vi "UI_Template_modify.vi"() -> ()   [LabVIEW 2014]
uses:
  Terminal_Global_Template_Name.vi
panel:
  in  "退出":bool
  in  "模板名称 2":string
  out "tempNo":string
  in  "修改载荷谱模板 2":string[][](table)
  in  "模板名称":string
  in  "保存修改":bool
  in  "修改载荷谱模板":string[][](table)
  # "载荷谱模板修改"
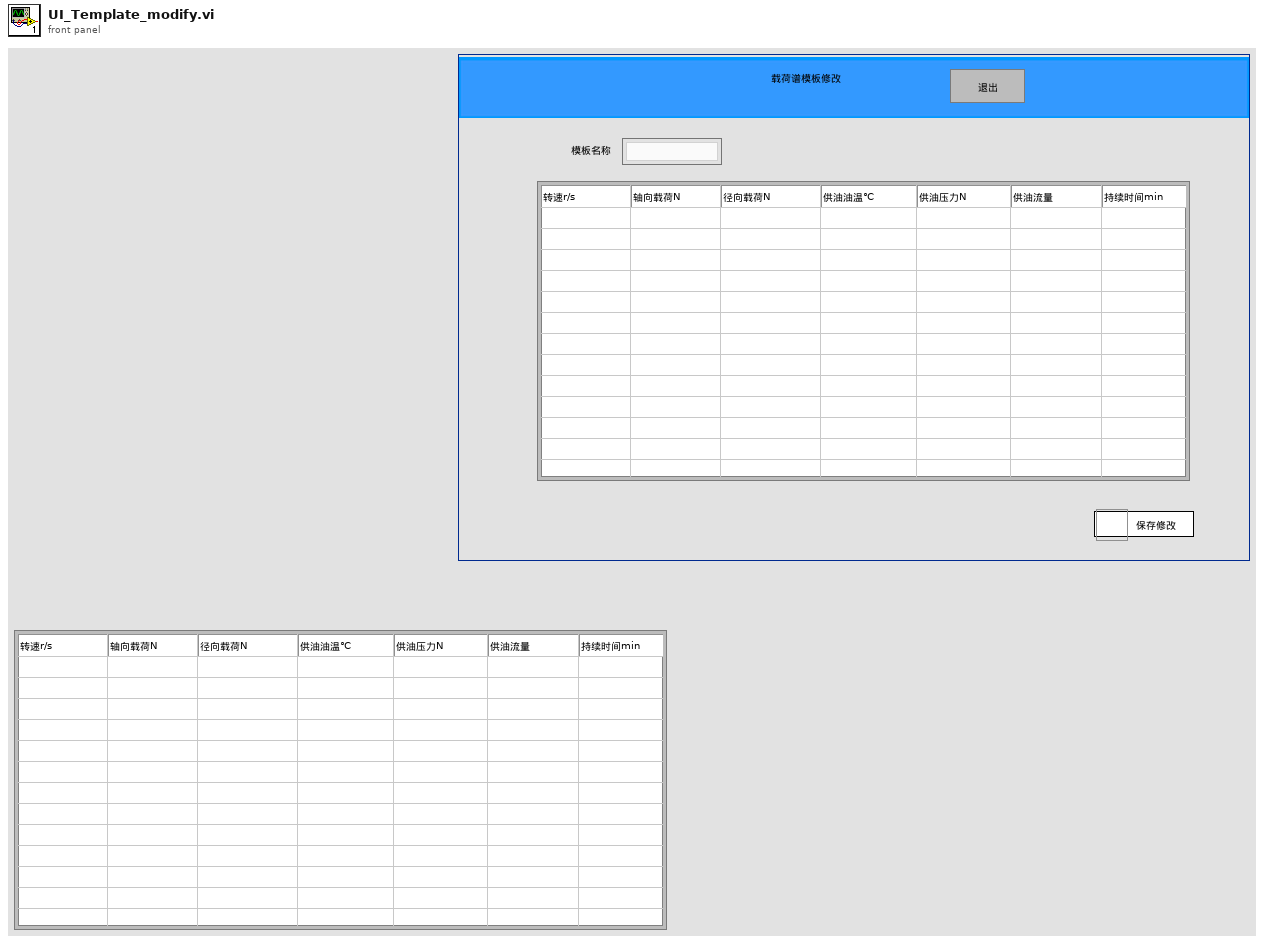
[diagram p1: front panel]
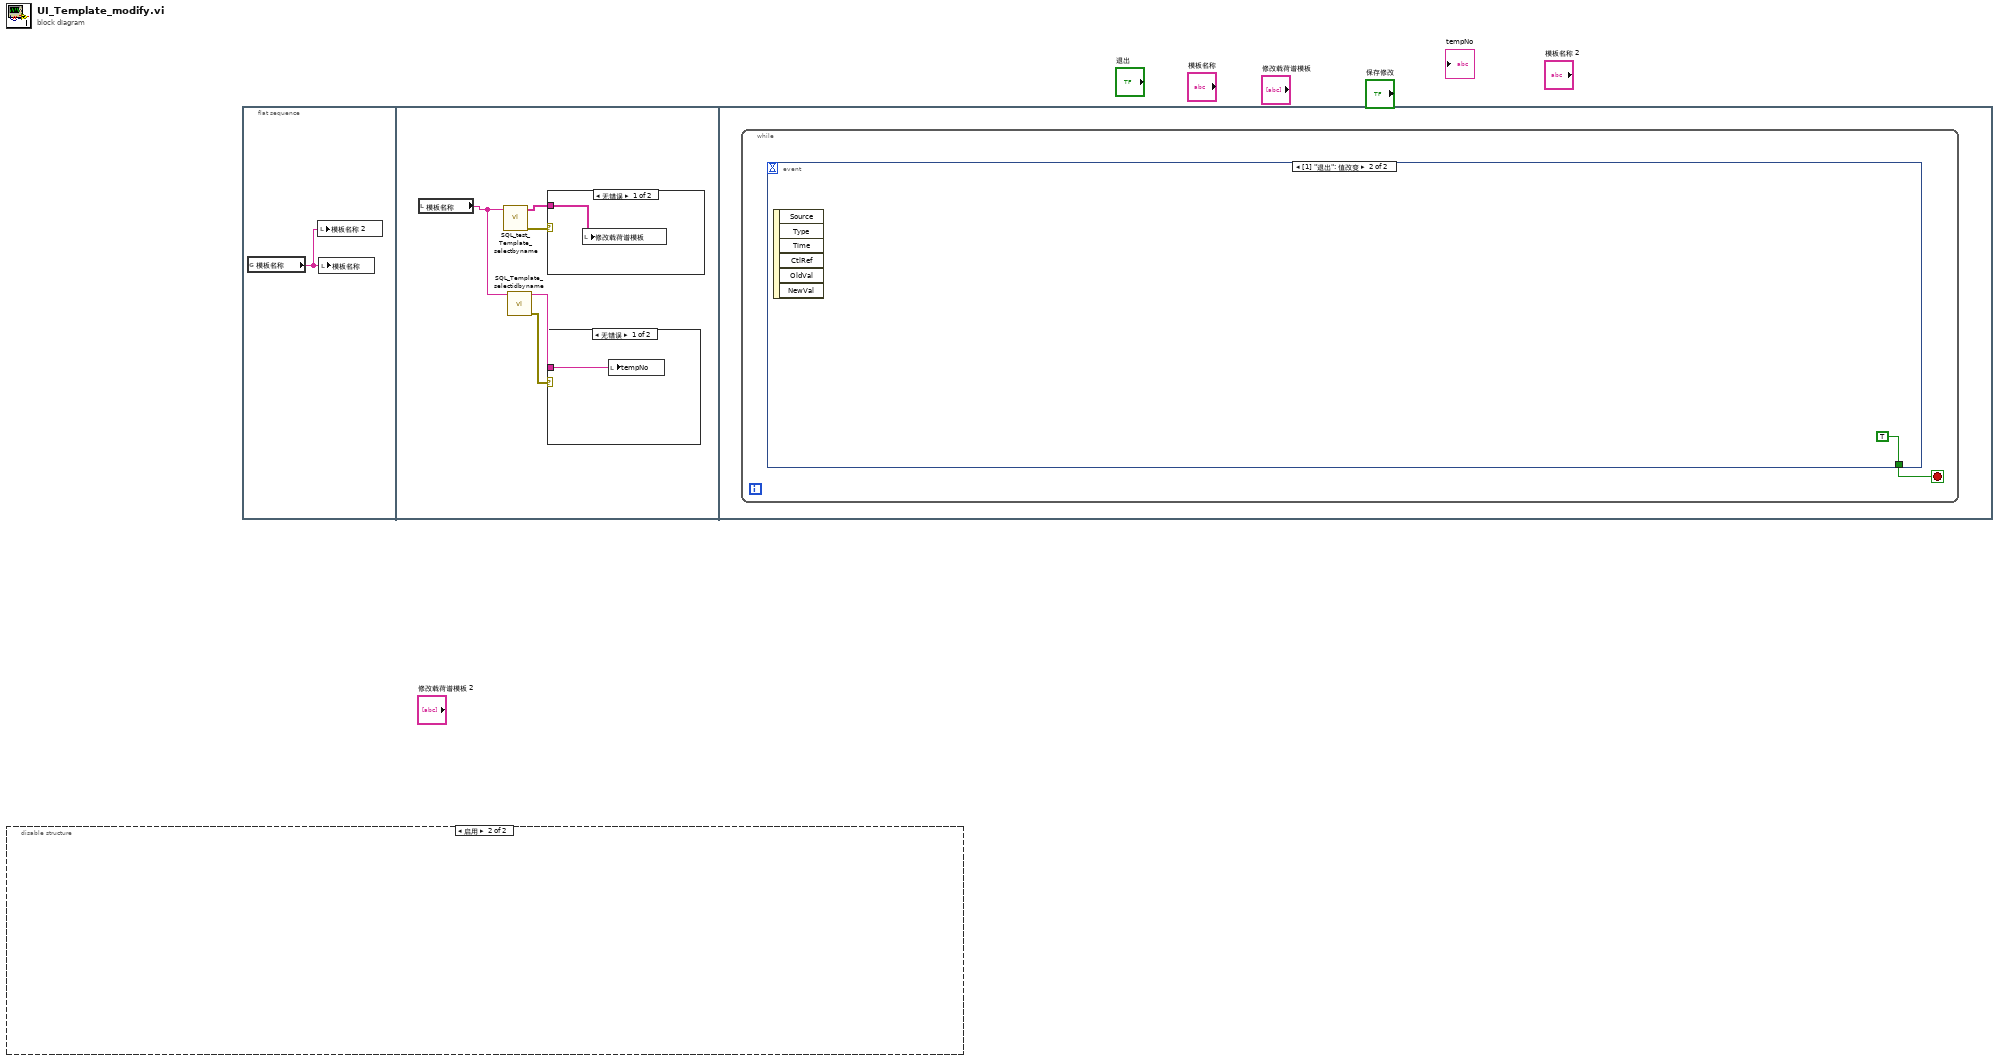
[diagram p0: block diagram]
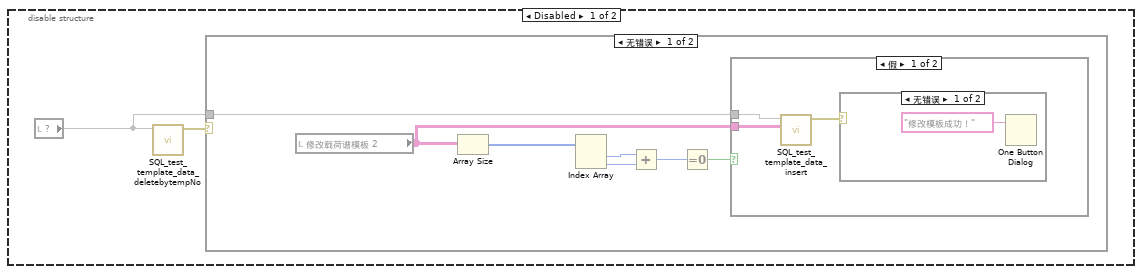
[diagram p2: hidden frame]
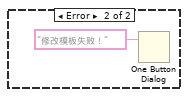
[diagram p3: hidden frame]
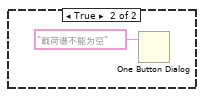
[diagram p4: hidden frame]
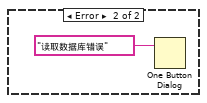
[diagram p6: hidden frame]
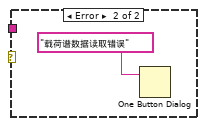
[diagram p7: hidden frame]
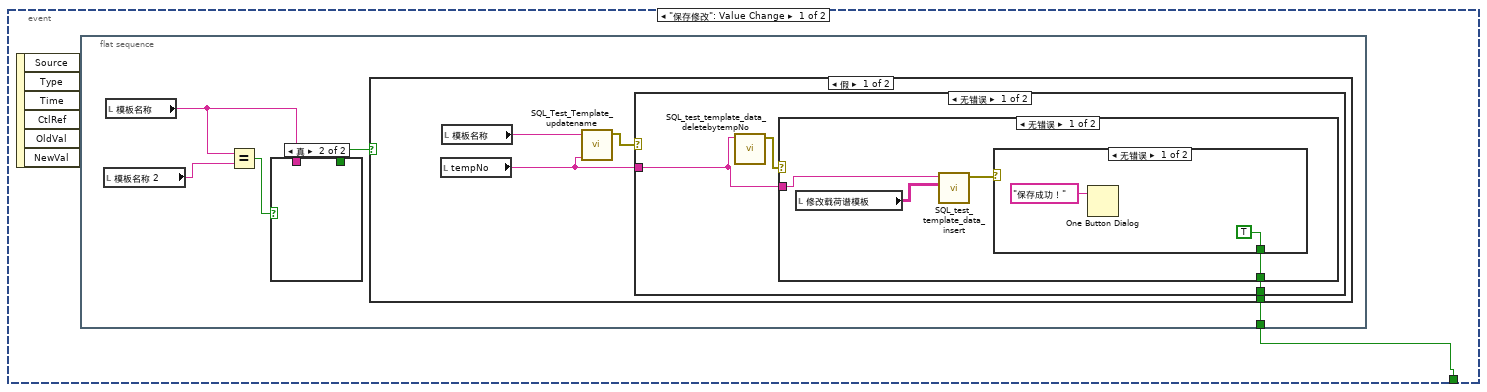
[diagram p8: hidden frame]
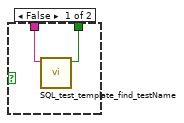
[diagram p9: hidden frame]
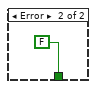
[diagram p10: hidden frame]
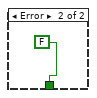
[diagram p11: hidden frame]
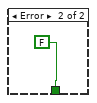
[diagram p12: hidden frame]
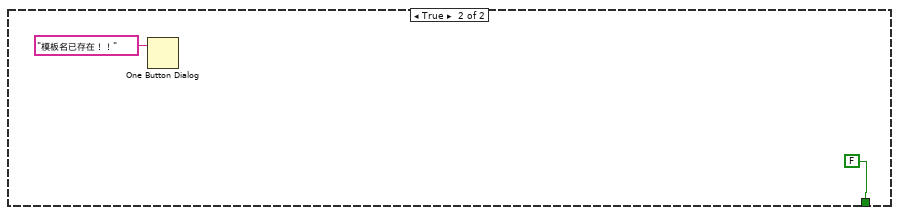
[diagram p13: hidden frame]
diagram:
  n1 = disable-structure shown="启用" {
    frame Disabled {
      n2 = local read item#-1() -> (w1)
      n3 = call "SQL_test_template_data_deletebytempNo.vi"("tempNo"=w1) -> ("error out"=w2:errorcluster)  [unwired: 10 in]
      n4 = case shown="无错误" w2 {
        tunnel: w1 -> [w3 _]
        frame No Error {
          n5 = local read "修改载荷谱模板 2"() -> (w4:string[][])
          n6 = Array Size(array=w4) -> (size(s)=w9:i32[])
          n7 = Index Array(array=w9) -> (element #1=w8:i32, element #2=w7:i32)  [unwired: 2 in]
          n8 = Add(x=w8, y=w7) -> (x+y=w6:i32)
          n9 = Equal To 0?(x=w6) -> (x = 0?=w5:bool)
          n10 = case shown="假" w5 {
            tunnel: w4 -> [w11 _]
            tunnel: w3 -> [w10 _]
            frame False {
              n11 = call "SQL_test_template_data_insert.vi"("表格控件"=w11, "tempNo"=w10) -> ("error out"=w12:errorcluster)  [unwired: 9 in]
              n12 = case shown="无错误" w12 {
                frame No Error {
                  n13 = One Button Dialog(message="修改模板成功！" ("消息")) -> ()  [unwired: 1 in, 1 out]
                }
                frame Error {
                  n14 = One Button Dialog(message="修改模板失败！" ("消息")) -> ()  [unwired: 1 in, 1 out]
                }
              }
            }
            frame True {
              n15 = One Button Dialog(message="载荷谱不能为空" ("消息")) -> ()  [unwired: 1 in, 1 out]
            }
          }
        }
        frame Error {
        }
      }
    }
    frame Enabled {
    }
  }
  n16 = flat-sequence {
    frame #0 {
      n17 = global read "Terminal_Global_Template_Name.vi" "模板名称"() -> (w16:string)
      n18 = local write "模板名称 2"(w16) -> ()
      n19 = local write "模板名称"(w16) -> ()
    }
    frame #1 {
      n20 = local read "模板名称"() -> (w21:string)
      n21 = call "SQL_test_Template_selectbyname.vi"("模板名称"=w21) -> ("error out"=w20:errorcluster, "载荷谱信息"=w19:string[][])  [unwired: 9 in]
      n22 = call "SQL_Template_selectidbyname.vi"("模板名称"=w21) -> ("error out"=w18:errorcluster, "tempNo"=w17:string)  [unwired: 9 in]
      n23 = case shown="无错误" w20 {
        tunnel: w19 -> [w24 _]
        frame No Error {
          n24 = local write "修改载荷谱模板"(w24) -> ()
        }
        frame Error {
          n25 = One Button Dialog(message="载荷谱数据读取错误" ("消息")) -> ()  [unwired: 1 in, 1 out]
        }
      }
      n26 = case shown="无错误" w18 {
        tunnel: w17 -> [w22 _]
        frame No Error {
          n27 = local write "tempNo"(w22) -> ()
        }
        frame Error {
          n28 = One Button Dialog(message="读取数据库错误" ("消息")) -> ()  [unwired: 1 in, 1 out]
        }
      }
    }
    frame #2 {
      n29 = while {
        stop <- w26 stop-if-true
        n30 = event shown="[1] \"退出\": 值改变" {
          selector: _ -> [_ _]
          dyn-events: _ -> [_ _]
          timeout: _ -> [_ _]
          tunnel: [w27 TRUE] -> w26
          event "保存修改": Value Change {
            n31 = event-data() -> ()  [unwired: 1 in, 6 out]
            n32 = flat-sequence {
              tunnel: [w32] -> w27
              frame #0 {
                n33 = local read "模板名称 2"() -> (w31:string)
                n34 = local read "模板名称"() -> (w29:string)
                n35 = Equal?(x=w29, y=w31) -> (x = y?=w30:bool)
                n36 = case shown="真" w30 {
                  tunnel: w29 -> [w34 _]
                  tunnel: [w33 _] -> w28
                  frame False {
                    n37 = call "SQL_test_template_find_testName.vi"("模板名称"=w34) -> ("模板是否存在"=w33:bool)  [unwired: 10 in]
                  }
                  frame True {
                  }
                }
                n38 = case shown="假" w28 {
                  tunnel: [w35 FALSE] -> w32
                  frame False {
                    n39 = local read "tempNo"() -> (w36:string)
                    n40 = local read "模板名称"() -> (w38:string)
                    n41 = call "SQL_Test_Template_updatename.vi"("tempNo"=w36, "tempName"=w38) -> ("error out"=w37:errorcluster)  [unwired: 9 in]
                    n42 = case shown="无错误" w37 {
                      tunnel: w36 -> [w40 _]
                      tunnel: [w39 FALSE] -> w35
                      frame No Error {
                        n43 = call "SQL_test_template_data_deletebytempNo.vi"("tempNo"=w40) -> ("error out"=w41:errorcluster)  [unwired: 10 in]
                        n44 = case shown="无错误" w41 {
                          tunnel: w40 -> [w45 _]
                          tunnel: [w42 FALSE] -> w39
                          frame No Error {
                            n45 = local read "修改载荷谱模板"() -> (w44:string[][])
                            n46 = call "SQL_test_template_data_insert.vi"("表格控件"=w44, "tempNo"=w45) -> ("error out"=w43:errorcluster)  [unwired: 9 in]
                            n47 = case shown="无错误" w43 {
                              tunnel: [TRUE FALSE] -> w42
                              frame No Error {
                                n48 = One Button Dialog(message="保存成功！" ("消息")) -> ()  [unwired: 1 in, 1 out]
                              }
                              frame Error {
                              }
                            }
                          }
                          frame Error {
                          }
                        }
                      }
                      frame Error {
                      }
                    }
                  }
                  frame True {
                    n49 = One Button Dialog(message="模板名已存在！！" ("消息")) -> ()  [unwired: 1 in, 1 out]
                  }
                }
              }
            }
          }
          event "退出": Value Change {
            n50 = event-data() -> ()  [unwired: 1 in, 6 out]
          }
        }
      }
    }
  }
